vi "Message Packet Decoding.vi"(8 "error in (no error)":errorcluster, 10 "Data":string, 11 "HSMS Class in":refnum<class "HSMS Class.lvclass">) -> (0 "error out":errorcluster, 2 "Message Packet":T1, 3 "HSMS Class out":refnum<class "HSMS Class.lvclass">)   [LabVIEW 2020, in "SECS Communication.lvlib" / "HSMS Class.lvclass"]
uses:
  HSMS Class.lvclass
  Message Packet.ctl
  Message Header.ctl
  PType.ctl
  SType.ctl
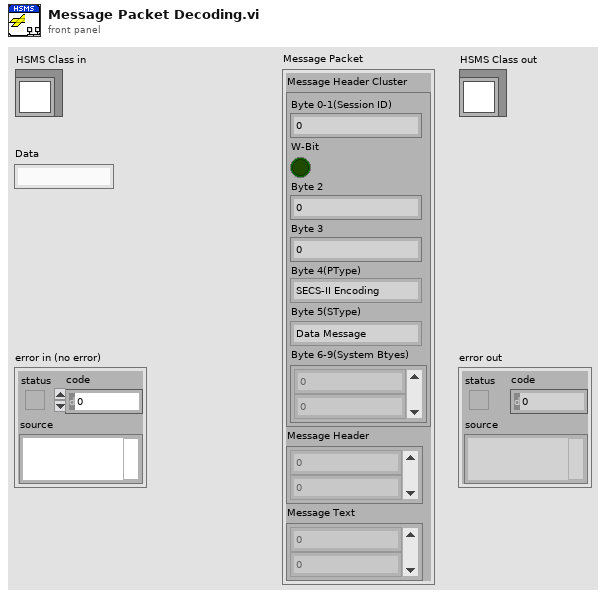
[diagram p1: front panel]
types:
  T1 = typedef "SECS Communication.lvlib/HSMS Class.lvclass/Message Packet.ctl" = cluster{"Message Header Cluster":T2, "Message Header":u8[], "Message Text":u8[]}
  T2 = typedef "SECS Communication.lvlib/HSMS Class.lvclass/Message Header.ctl" = cluster{"Byte 0-1(Session ID)":u16, "W-Bit":bool, "Byte 2":u8, "Byte 3":u8, "Byte 4(PType)":T3, "Byte 5(SType)":T4, "Byte 6-9(System Btyes)":u8[]}
  T3 = typedef "SECS Communication.lvlib/HSMS Class.lvclass/PType.ctl" = enum8{"SECS-II Encoding", "Reserved"}
  T4 = typedef "SECS Communication.lvlib/HSMS Class.lvclass/SType.ctl" = enum8{"Data Message", "Select.req", "Select.rsp", "Deselect.req", "Deselect.rsp", "Linktest.req", "Linktest.rsp", "Reject.req", "Separate.req"}
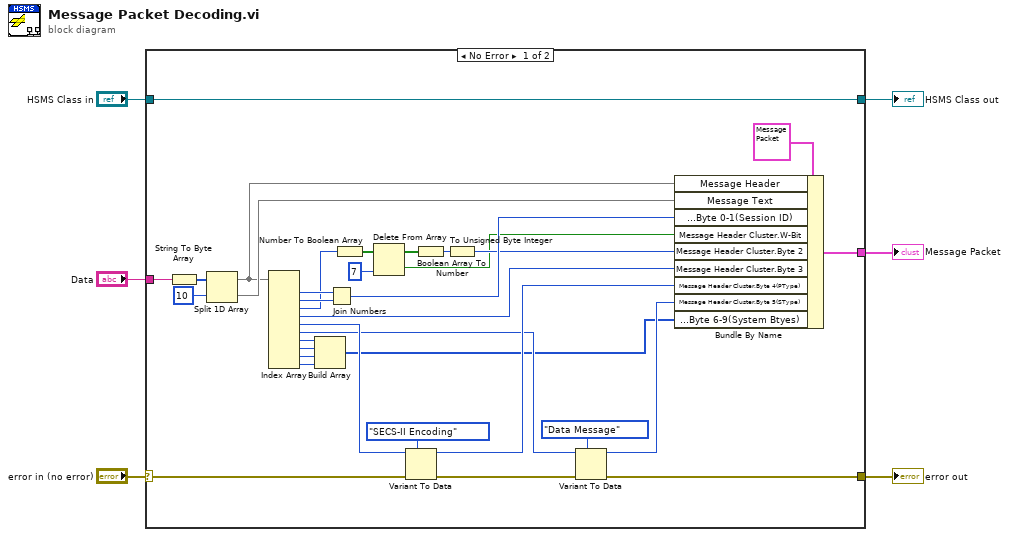
[diagram p0: block diagram]
diagram:
  n1 = case shown="No Error" "error in (no error)" {
    selector: "error in (no error)" -> [w24 w41]
    tunnel: [w12 _] -> w4
    tunnel: "Data" -> [w14 _]
    tunnel: "HSMS Class in" -> [w13 w40]
    tunnel: [w13 w40] -> w1
    tunnel: [w11 w41] -> w2
    frame No Error {
      n2 = String To Byte Array(string=w14) -> (unsigned byte array=w37:u8[])
      n3 = Split 1D Array(array=w37, index=10) -> (first subarray=w10:u8[], second subarray=w15:u8[])
      n4 = Index Array(array=w10) -> (element #1=w39:u8, element #2=w38:u8, element #3=w30:u8, element #4=w25:u8, element #5=w23:u8, element #6=w19:u8, element #7=w35:u8, element #8=w36:u8, element #9=w34:u8, element #10=w33:u8)  [unwired: 10 in]
      n5 = Build Array(w35, w36, w34, w33) -> (w16:u8[])
      n6 = Join Numbers(hi=w39, lo=w38) -> ((hi.lo)=w27:u16)
      n7 = Number To Boolean Array(number=w30) -> (Boolean array=w9:bool[])
      n8 = Delete From Array(array=w9, index=7) -> (deleted portion=w7:bool, array with subset deleted=w29:bool[])  [unwired: 1 in]
      n9 = Variant To Data(error in=w24, type=PType."SECS-II Encoding" ("Byte 4(PType)"), Variant=w23) -> (data=w21:T3, error out=w20:errorcluster)
      n10 = Boolean Array To Number(Boolean array=w29) -> (number=w31:u32)
      n11 = To Unsigned Byte Integer(number=w31) -> (unsigned 8bit integer=w26:u8)
      n12 = Variant To Data(error in=w20, type=SType."Data Message" ("Byte 5(SType)"), Variant=w19) -> (data=w17:T4, error out=w11:errorcluster)
      n13 = Bundle By Name(cluster=T1 {"Message Header Cluster"={"Byte 0-1(Session ID)"=0, "W-Bit"=FALSE, "Byte 2"=0, "Byte 3"=0, "Byte 4(PType)"=enum."SECS-II Encoding", "Byte 5(SType)"=enum."Data Message", "Byte 6-9(System Btyes)"=[]}, "Message Header"=[], "Message Text"=[]} ("Message Packet"), "Message Header"=w10, "Message Text"=w15, "Message Header Cluster.Byte 0-1(Session ID)"=w27, "Message Header Cluster.W-Bit"=w7, "Message Header Cluster.Byte 2"=w26, "Message Header Cluster.Byte 3"=w25, "Message Header Cluster.Byte 4(PType)"=w21, "Message Header Cluster.Byte 5(SType)"=w17, "Message Header Cluster.Byte 6-9(System Btyes)"=w16) -> (w12:T1)
    }
    frame Error {
    }
  }
  "error out" <- w2
  "Message Packet" <- w4
  "HSMS Class out" <- w1
